vi "Core.vi"(11 "Module in":refnum<class "Module.lvclass">) -> ()   [LabVIEW 2020, in "Module.lvclass"]
doc: "This template is for the Queued Message Handler design pattern.\n\nThe Event Handling Loop generates messages based on user interface actions.\n\nThe Message Handling Loop processes messages generated by the Event Handling Loop, or by other messages. The messages are string values, so new messages can be added easily to the Message Cases case structure in the Message Handling Loop. Each message cluster can also provide an optional value for Message Data, which is a variant that can be converted to whatever message-specific data is required."
uses:
  Module.lvclass
  <vilib>/Utility/error.llb/Error Cluster From Error Code.vi
  <vilib>/ErrorRing/Error Ring.xnode
  <vilib>/NI_Real-Time Target Support.lvlib
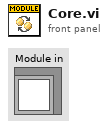
[diagram p1: front panel]
types:
  T1 = enum32{"Invalid", "Standard", "Closed", "Hidden", "Minimized", "Maximized"}
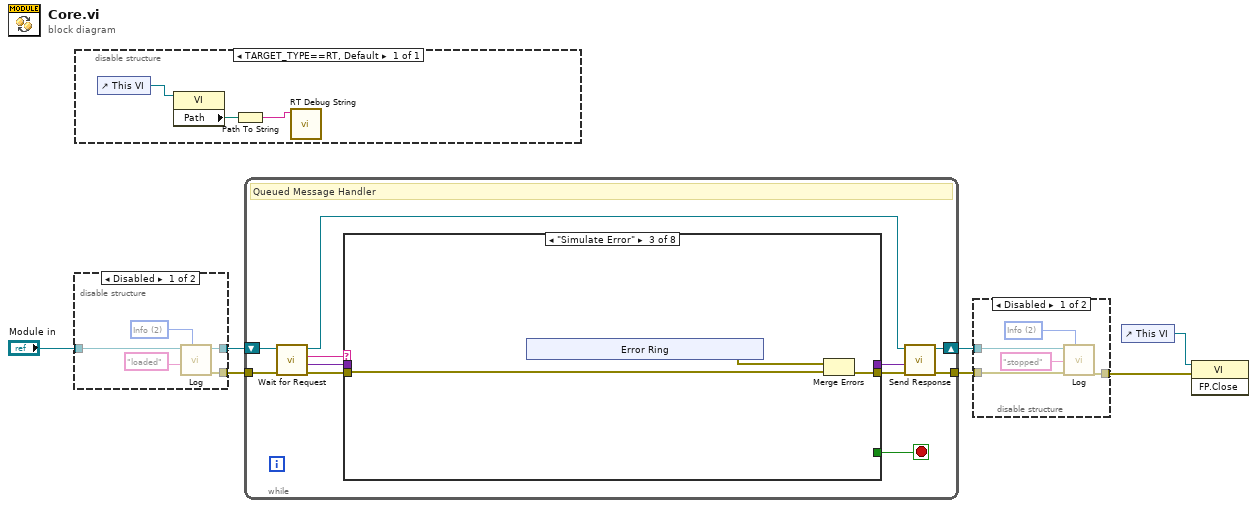
[diagram p0: block diagram]
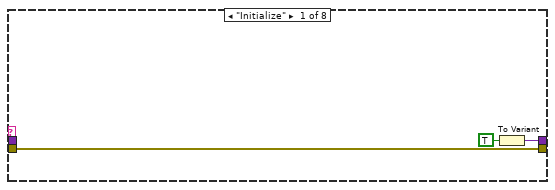
[diagram p2: hidden frame]
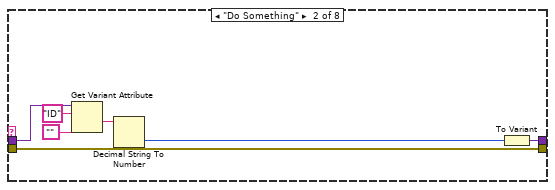
[diagram p3: hidden frame]
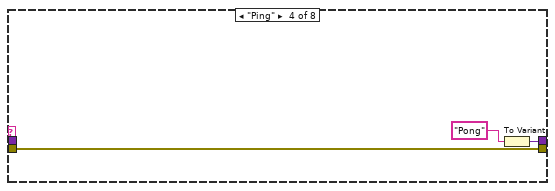
[diagram p4: hidden frame]
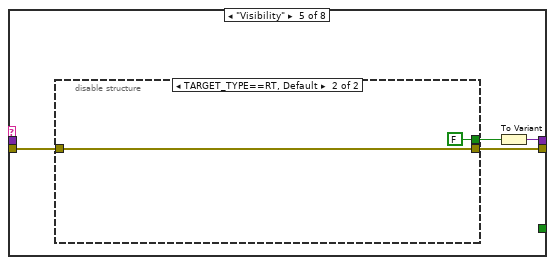
[diagram p5: hidden frame]
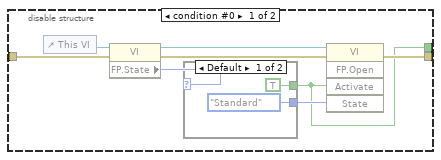
[diagram p6: hidden frame]
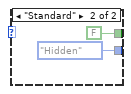
[diagram p7: hidden frame]
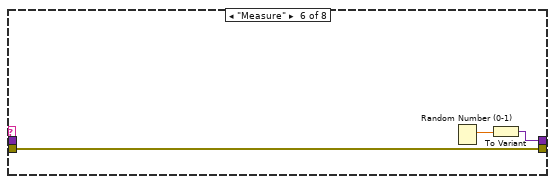
[diagram p8: hidden frame]
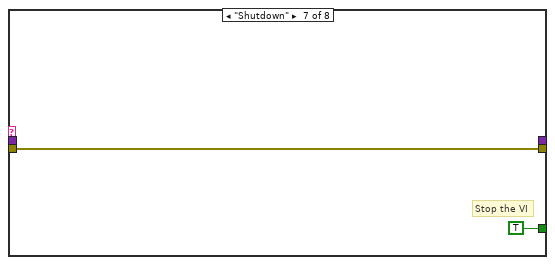
[diagram p9: hidden frame]
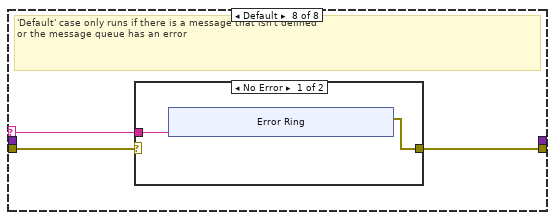
[diagram p10: hidden frame]
diagram:
  n1 = disable-structure shown="Disabled" {
    disable-tunnel: [w11 w13] -> w7
    disable-tunnel: "Module in" -> [w10 w13]
    disable-tunnel: [w9 _] -> w5
    frame Disabled {
      w8 = 2 items=["Error", "Warning", "Info"] ("severity")
      n2 = call "Log.vi"("severity"=w8, "Data"="loaded" ("Originator"), "Module in"=w10) -> ("error out"=w9:errorcluster, "Module out"=w11:refnum<class "Module.lvclass">)  [unwired: 7 in]
    }
    frame Enabled {
    }
  }
  n3 = disable-structure shown="TARGET_TYPE==RT, Default" {
    frame condition #0 (active) {
      n4 = control-ref of="This VI"() -> (w16:refnum<vi>)
      n5 = property class="VI"(reference=w16) -> ("Path"=w15:path)  [unwired: 1 in, 2 out]
      n6 = Path To String(path=w15) -> (string=w14:string)
      n7 = call <vilib>:"RT Debug String.vi"("String to write"=w14) -> ()  [unwired: 10 in, 1 out]
    }
  }
  n8 = while {
    shift-right: [w27] -> w4
    shift-left: w7 -> [w23]
    tunnel: w5 -> [w21]
    tunnel: [w24] -> w1
    stop <- w22 stop-if-true
    # "Queued Message Handler"
    n9 = call "Wait for Request.vi"("error in"=w21, "Module in"=w23) -> ("error out"=w20:errorcluster, "Data"=w19:variant, "Message"=w18:string, "Module out"=w17:refnum<class "Module.lvclass">)  [unwired: 6 in]
    n10 = case shown="\"Simulate Error\"" w18 {
      selector: w18 -> [_ _ _ _ _ _ _ w73]
      tunnel: w20 -> [w28 w33 w39 w48 w52 w69 w70 w74]
      tunnel: [_ _ _ _ _ _ TRUE _] -> w22
      tunnel: w19 -> [_ w34 _ _ _ _ _ _]
      tunnel: [w30 w32 _ w47 w50 w68 _ _] -> w26
      tunnel: [w28 w33 w40 w48 w51 w69 w70 w72] -> w25
      frame "Initialize" {
        n11 = To Variant(anything=TRUE) -> (Variant=w30:variant)
      }
      frame "Do Something" {
        n12 = Get Variant Attribute(Variant=w34, name="ID", default value (empty Variant)="") -> (value=w35:string)  [unwired: 1 in, 3 out]
        n13 = Decimal String To Number(string=w35) -> (number=w31:i32)  [unwired: 2 in, 1 out]
        n14 = To Variant(anything=w31) -> (Variant=w32:variant)
      }
      frame "Simulate Error" {
        n15 = xnode "Error Ring"() -> ("error out"=w38:errorcluster)
        n16 = Merge Errors(w38, w39) -> (w40:errorcluster)
      }
      frame "Ping" {
        n17 = To Variant(anything="Pong") -> (Variant=w47:variant)
      }
      frame "Visibility" {
        n18 = disable-structure shown="TARGET_TYPE==RT, Default" {
          disable-tunnel: w52 -> [w60 w66]
          disable-tunnel: [w54 w66] -> w51
          disable-tunnel: [w53 FALSE ("Activate?")] -> w49
          frame condition #0 {
            n19 = control-ref of="This VI"() -> (w59:refnum<vi>)
            n20 = property class="VI"(reference=w59, error in=w60) -> (reference out=w57:refnum<vi>, error out=w58:errorcluster, "FP.State"=w56:T1)
            n21 = case shown="Default" w56 {
              tunnel: [T1."Standard" ("State") T1."Hidden" ("State")] -> w55
              tunnel: [TRUE ("Activate?") FALSE ("Activate?")] -> w53
              frame Default {
              }
              frame "Standard" {
              }
            }
            n22 = invoke class="VI" method="FP.Open"(reference=w57, error in=w58, "Activate"=w53, "State"=w55) -> (error out=w54:errorcluster)  [unwired: 1 in, 4 out]
          }
          frame condition #1 (active) {
          }
        }
        n23 = To Variant(anything=w49) -> (Variant=w50:variant)
      }
      frame "Measure" {
        n24 = Random Number (0-1)() -> (number: 0 to 1=w67:dbl)
        n25 = To Variant(anything=w67) -> (Variant=w68:variant)
      }
      frame "Shutdown" {
        # "Stop the VI"
      }
      frame Default {
        # "'Default' case only runs if there is a message that isn't defined\nor the message queue has an error"
        n26 = case shown="No Error" w74 {
          selector: w74 -> [_ w84]
          tunnel: w73 -> [w76 _]
          tunnel: [w75 w84] -> w72
          frame No Error {
            n27 = xnode ("Error Ring")("parameter 0"=w76) -> ("error out"=w75:errorcluster)
          }
          frame Error {
          }
        }
      }
    }
    n28 = call "Send Response.vi"("error in"=w25, "Response"=w26, "Module in"=w17) -> ("error out"=w24:errorcluster, "Module out"=w27:refnum<class "Module.lvclass">)  [unwired: 7 in]
  }
  n29 = disable-structure shown="Disabled" {
    disable-tunnel: w1 -> [w88 _]
    disable-tunnel: w4 -> [w87 _]
    disable-tunnel: [w86 _] -> w2
    frame Disabled {
      w85 = 2 items=["Error", "Warning", "Info"] ("severity")
      n30 = call "Log.vi"("severity"=w85, "error in (no error)"=w88, "Data"="stopped" ("Originator"), "Module in"=w87) -> ("error out"=w86:errorcluster)  [unwired: 6 in, 1 out]
    }
    frame Enabled {
    }
  }
  n31 = control-ref of="This VI"() -> (w3:refnum<vi>)
  n32 = invoke class="VI" method="FP.Close"(reference=w3, error in=w2) -> ()  [unwired: 1 in, 3 out]
